vi "flight_time_05_12.vi"() -> ()   [LabVIEW 2013]
uses:
  <vilib>/Instr/_visa.llb/VISA Configure Serial Port (Instr).vi
  <vilib>/Analysis/NI_AALBase.lvlib
panel:
  out "h":dbl
  out "calibrado3 2":dbl(graph) caption="Tempo de voo"
  in  "lock":u8
  out "avg_cell4":dbl
  out "avg_cell3":dbl
  out "avg_cell2":dbl
  out "avg_cell1":dbl
  in  "stop":bool
  in  "Pcell1":u32[](array[numeric])
  in  "Pcell2":u32[](array[numeric])
  in  "Pcell3":u32[](array[numeric])
  in  "Pcell4":u32[](array[numeric])
  out "time":u32[](graph)
  in  "Tab Control":enum32{"Calibração", "filter"}(tab)
  out "raw_cell1":i32(graph) caption="Celula 1"
  out "raw_cell2":i32(graph) caption="Celula 2"
  out "raw_cell3":i32(graph) caption="Celula 3"
  out "raw_cell4":i32(graph) caption="Celula 4"
  out "calibrado1":dbl(graph) caption="Celula 1"
  out "calibrado3":dbl(graph) caption="Celula 3"
  out "calibrado2":dbl(graph) caption="Celula 2"
  out "calibrado4":dbl(graph) caption="Celula 4"
  out "celula 7":dbl(graph)
  in  "?":bool
  out "tempo de voo (ms)":dbl
  out "stop 2":dbl
  out "start":dbl
  in  "?":bool
  out "cell":u8[](array[numeric])
  out "output_int16":i32[](array[numeric])
  out "data":u8[](array[numeric])
  in  "serial_port":refnum<visa-resource-name> caption="Porta Serial"
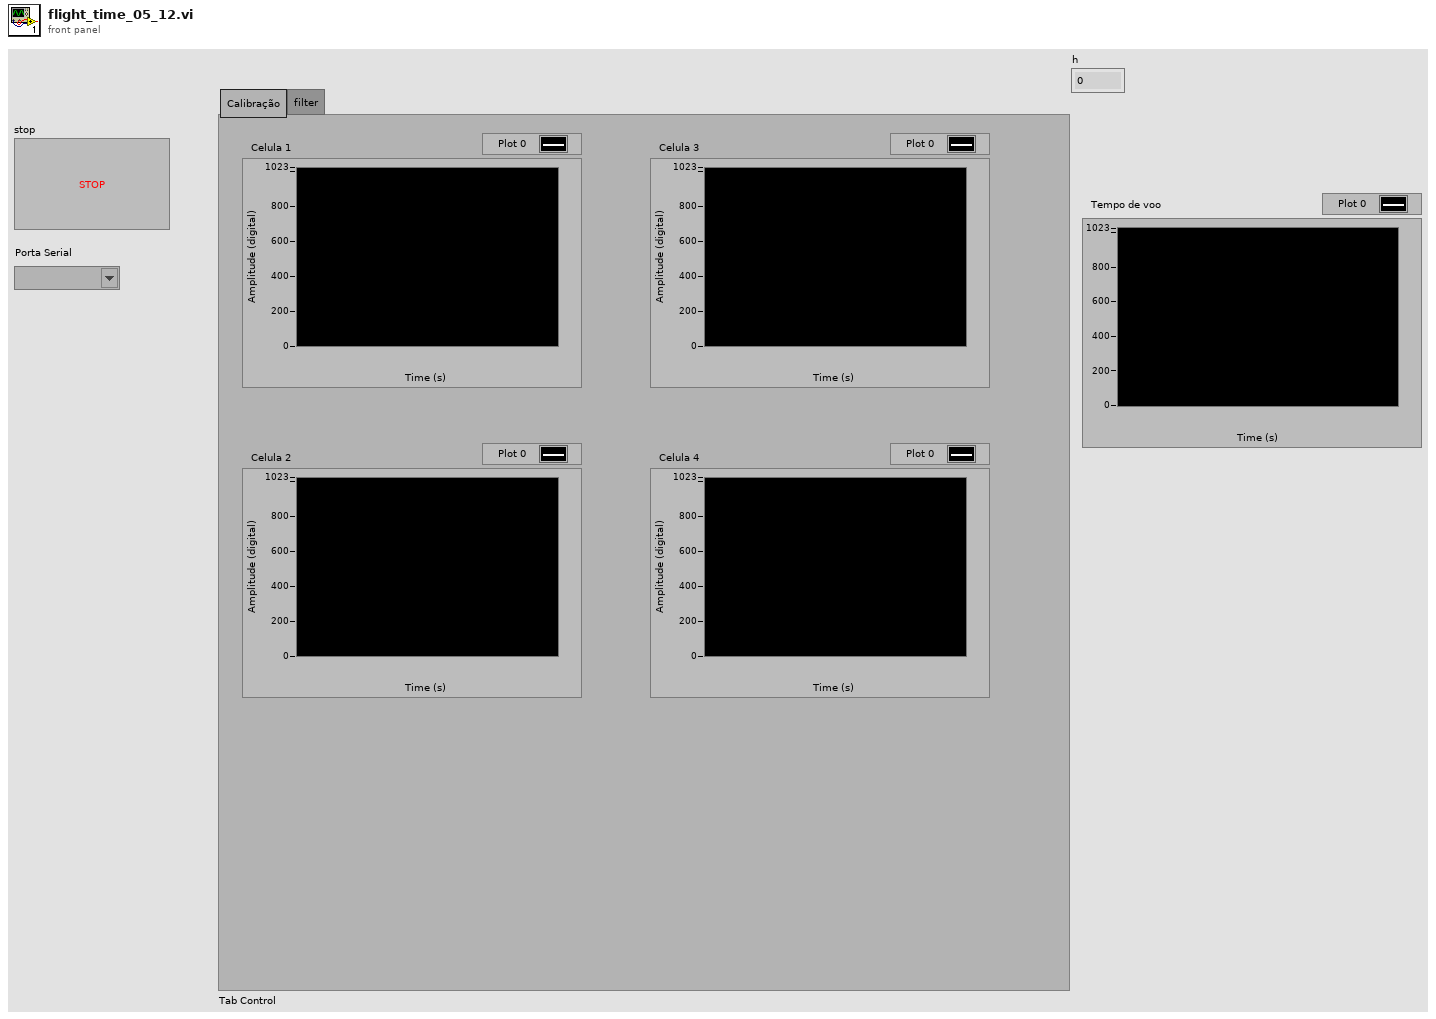
[diagram p1: front panel]
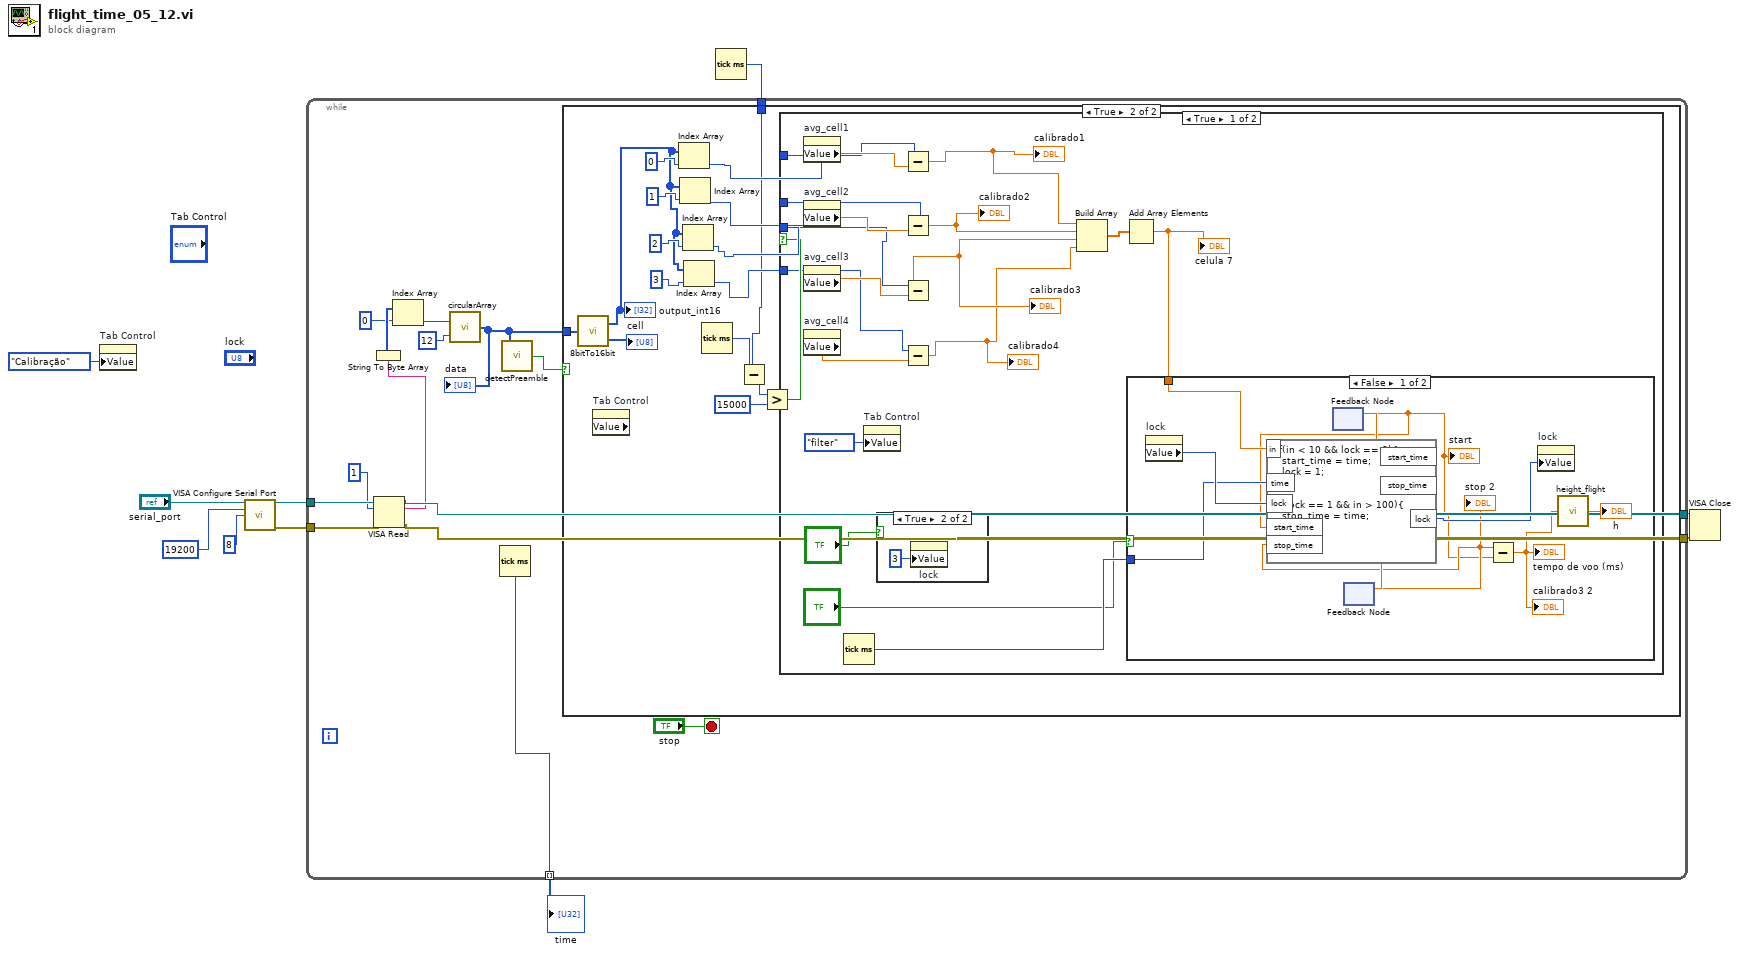
[diagram p0: block diagram]
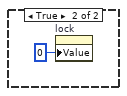
[diagram p4: hidden frame]
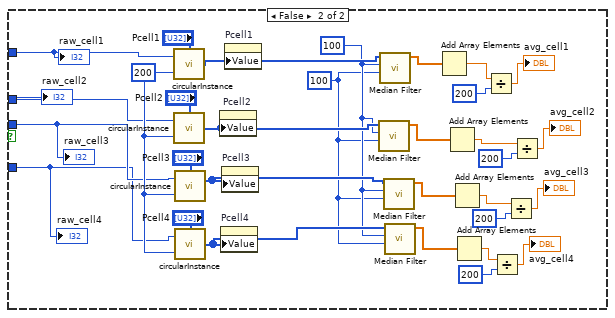
[diagram p5: hidden frame]
diagram:
  n1 = property on="Tab Control" class="TabCtl (strict)"("Value"=enum32{"Calibração", "filter"}."Calibração" ("Tab Control")) -> ()  [unwired: 2 in, 2 out]
  n2 = call-poly "VISA Configure Serial Port"("VISA resource name"="serial_port", "baud rate (9600)"=u32 19200, "data bits (8)"=u16 8) -> ("VISA resource name out"=w7:refnum<visa-resource-name>, "error out"=w6:errorcluster)  [unwired: 11 in]
  n3 = Tick Count (ms)() -> (millisecond timer value=w2:u32)
  n4 = while {
    tunnel: w7 -> [w25]
    tunnel: w6 -> [w24]
    tunnel: [w22] -> w4
    tunnel: [w23] -> w5
    tunnel: [w13] -> w3 mode=indexing
    tunnel: w2 -> [w11]
    stop <- "stop" stop-if-true
    n5 = VISA Read(VISA resource name=w25, byte count=1, error in (no error)=w24) -> (VISA resource name out=w23:refnum<visa-resource-name>, read buffer=w17:string, error out=w22:errorcluster)  [unwired: 1 out]
    n6 = String To Byte Array(string=w17) -> (unsigned byte array=w20:u8[])
    n7 = Index Array(array=w20, index=0) -> (element=w14:u8)
    n8 = call "circularArray.vi"("max-size"=u8 12, "element"=w14) -> ("dataout"=w15:u8[])
    "data" <- w15
    n9 = Tick Count (ms)() -> (millisecond timer value=w13:u32)
    n10 = call "detectPreamble.vi"("data-in"=w15) -> ("detected"=w12:bool)
    n11 = case shown="True" w12 {
      tunnel: w15 -> [_ w40]
      tunnel: w11 -> [_ w29]
      frame False {
      }
      frame True {
        n12 = call "8bitTo16bit.vi"("input_byte"=w40) -> ("output_int16"=w35:i32[], "cell"=→"cell":u8[])
        "output_int16" <- w35
        n13 = property on="Tab Control" class="TabCtl (strict)" props=["Value"]() -> ()  [unwired: 2 in, 3 out]
        n14 = Index Array(array=w35, index=0) -> (element=w31:i32)
        n15 = Index Array(array=w35, index=1) -> (element=w32:i32)
        n16 = Index Array(array=w35, index=2) -> (element=w33:i32)
        n17 = Index Array(array=w35, index=3) -> (element=w34:i32)
        n18 = Tick Count (ms)() -> (millisecond timer value=w30:u32)
        n19 = Subtract(x=w30, y=w29) -> (x-y=w28:u32)
        n20 = Greater?(x=w28, y=u32 15000) -> (0:w26:bool)
        n21 = case shown="True" w26 {
          tunnel: w31 -> [w51 w75]
          tunnel: w32 -> [w48 w74]
          tunnel: w33 -> [w49 w73]
          tunnel: w34 -> [w50 w72]
          frame True {
            n22 = property on="avg_cell1" class="DigNum (strict)"() -> ("Value"=w57:dbl)  [unwired: 2 in, 2 out]
            n23 = property on="avg_cell2" class="DigNum (strict)"() -> ("Value"=w56:dbl)  [unwired: 2 in, 2 out]
            n24 = property on="avg_cell3" class="DigNum (strict)"() -> ("Value"=w55:dbl)  [unwired: 2 in, 2 out]
            n25 = property on="avg_cell4" class="DigNum (strict)"() -> ("Value"=w54:dbl)  [unwired: 2 in, 2 out]
            n26 = Tick Count (ms)() -> (millisecond timer value=w59:u32)
            n27 = property on="Tab Control" class="TabCtl (strict)"("Value"=enum32{"Calibração", "filter"}."filter" ("Tab Control")) -> ()  [unwired: 2 in, 2 out]
            n28 = case shown="True" "?" {
              frame False {
              }
              frame True {
                n29 = property on="lock" class="DigNum (strict)"("Value"=u8 3 ("lock")) -> ()  [unwired: 2 in, 2 out]
              }
            }
            n30 = Subtract(x=w51, y=w57) -> (x-y=w47:dbl)
            "calibrado1" <- w47
            n31 = Subtract(x=w48, y=w56) -> (x-y=w46:dbl)
            "calibrado2" <- w46
            n32 = Subtract(x=w49, y=w55) -> (x-y=w45:dbl)
            "calibrado3" <- w45
            n33 = Subtract(x=w50, y=w54) -> (x-y=w44:dbl)
            "calibrado4" <- w44
            n34 = Build Array(w47, w46, w45, w44) -> (w53:dbl[])
            n35 = Add Array Elements(numeric array=w53) -> (sum=w52:dbl)
            "celula 7" <- w52
            n36 = case shown="False" "?" {
              tunnel: w59 -> [w69 _]
              tunnel: w52 -> [w68 _]
              frame False {
                n37 = property on="lock" class="DigNum (strict)"() -> ("Value"=w70:u8)  [unwired: 2 in, 2 out]
                n38 = feedback #1() -> (w63:dbl)  [unwired: 1 in]
                "start" <- w63
                n39 = feedback #2() -> (w65:dbl)  [unwired: 1 in]
                "stop 2" <- w65
                n40 = formula code="if(in < 10 && lock == 0){\n  start_time = time;\n  lock = 1;\n}\n\nif(lock == 1 && in > 100){\n  stop_time = time;\n  lock = 0;\n}"("in"=w68, "time"=w69, "lock"=w70, "start_time"=w63, "stop_time"=w65) -> ("start_time"=w64:dbl, "stop_time"=w66:dbl, "lock"=w67:u8)
                n41 = feedback-in #1(w64) -> ()
                n42 = feedback-in #2(w66) -> ()
                n43 = Subtract(x=w65, y=w63) -> (x-y=w62:dbl)
                "tempo de voo (ms)" <- w62
                "calibrado3 2" <- w62
                n44 = property on="lock" class="DigNum (strict)"("Value"=w67) -> ()  [unwired: 2 in, 2 out]
                n45 = call "height_flight.vi"("t"=w62) -> ("h"=→"h":dbl)
              }
              frame True {
                n46 = property on="lock" class="DigNum (strict)"("Value"=u8 0 ("input variable")) -> ()  [unwired: 2 in, 2 out]
              }
            }
          }
          frame False {
            w92 = 100 ("left rank")
            w93 = 100 ("left rank")
            w100 = i16 200 ("max-size")
            n47 = call "circularInstance.vi"("data"="Pcell1", "max-size"=w100, "element"=w75) -> ("dataout"=w97:u32[])
            n48 = call "circularInstance.vi"("data"="Pcell2", "max-size"=w100, "element"=w74) -> ("dataout"=w96:u32[])
            n49 = call "circularInstance.vi"("data"="Pcell3", "max-size"=w100, "element"=w73) -> ("dataout"=w95:u32[])
            n50 = call "circularInstance.vi"("data"="Pcell4", "max-size"=w100, "element"=w72) -> ("dataout"=w94:u32[])
            n51 = property on="Pcell2" class="Arr (strict)"("Value"=w96) -> ()  [unwired: 2 in, 2 out]
            n52 = property on="Pcell4" class="Arr (strict)"("Value"=w94) -> ()  [unwired: 2 in, 2 out]
            n53 = property on="Pcell3" class="Arr (strict)"("Value"=w95) -> ()  [unwired: 2 in, 2 out]
            n54 = property on="Pcell1" class="Arr (strict)"("Value"=w97) -> ()  [unwired: 2 in, 2 out]
            n55 = call <vilib>:"Median Filter.vi"("right rank"=w92, "left rank"=w93, "X"=w96) -> ("Filtered X"=w91:dbl[])  [unwired: 7 in, 1 out]
            n56 = call <vilib>:"Median Filter.vi"("right rank"=w92, "left rank"=w93, "X"=w97) -> ("Filtered X"=w77:dbl[])  [unwired: 7 in, 1 out]
            n57 = call <vilib>:"Median Filter.vi"("right rank"=w92, "left rank"=w93, "X"=w95) -> ("Filtered X"=w90:dbl[])  [unwired: 7 in, 1 out]
            n58 = call <vilib>:"Median Filter.vi"("right rank"=w92, "left rank"=w93, "X"=w94) -> ("Filtered X"=w76:dbl[])  [unwired: 7 in, 1 out]
            n59 = Add Array Elements(numeric array=w77) -> (sum=w88:dbl)
            n60 = Add Array Elements(numeric array=w91) -> (sum=w78:dbl)
            n61 = Add Array Elements(numeric array=w90) -> (sum=w79:dbl)
            n62 = Add Array Elements(numeric array=w76) -> (sum=w80:dbl)
            n63 = Divide(x=w88, y=i16 200 ("max-size")) -> (x/y=→"avg_cell1":dbl)
            n64 = Divide(x=w80, y=i16 200 ("max-size")) -> (x/y=→"avg_cell4":dbl)
            n65 = Divide(x=w79, y=i16 200 ("max-size")) -> (x/y=→"avg_cell3":dbl)
            n66 = Divide(x=w78, y=i16 200 ("max-size")) -> (x/y=→"avg_cell2":dbl)
            "raw_cell1" <- w75
            "raw_cell2" <- w74
            "raw_cell3" <- w73
            "raw_cell4" <- w72
          }
        }
      }
    }
  }
  "time" <- w3
  n67 = VISA Close(VISA resource name=w5, error in (no error)=w4) -> ()  [unwired: 1 out]
